vi "4.3.vi"() -> ()   [LabVIEW 2017]
panel:
  out "平方根":dbl
  in  "数值":dbl
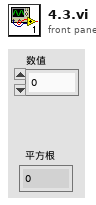
[diagram p1: front panel]
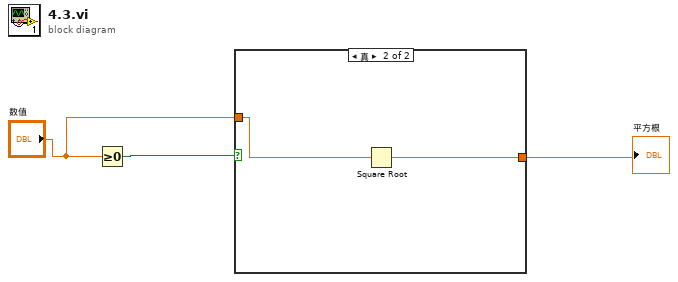
[diagram p0: block diagram]
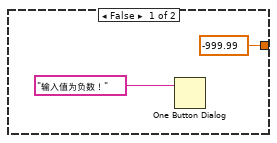
[diagram p2: hidden frame]
diagram:
  n1 = Greater Or Equal To 0?(x="数值") -> (x >= 0?=w3:bool)
  n2 = case shown="真" w3 {
    tunnel: "数值" -> [_ w7]
    tunnel: [-999.99 w6] -> w1
    frame False {
      n3 = One Button Dialog(message="输入值为负数！") -> ()  [unwired: 1 in, 1 out]
    }
    frame True {
      n4 = Square Root(x=w7) -> (sqrt(x)=w6:dbl)
    }
  }
  "平方根" <- w1
